vi "Package Typed Message.vi"(8 "error in (no error)":errorcluster, 11 "Group BOOL in":refnum<class "Group BOOL.lvclass">) -> (0 "error out":errorcluster, 2 "Data Msg":refnum<class "Message.lvclass">, 3 "Group BOOL out":refnum<class "Group BOOL.lvclass">)   [LabVIEW 2020, in "Vecto.lvlib" / "Group BOOL.lvclass"]
uses:
  Group BOOL.lvclass
  C:/dev/lv20CE/relink/lv-vecto/Vecto/Group/Group.lvclass
  lv-protoc/LV-Proto/Message/Message.lvclass
  Group/Group.lvclass/Group.ctl
  Group BOOL.lvclass/Group BOOL.ctl
  lv-volatus/messages/BoolData/Data.ctl
  Group Config/Group Config.lvclass/Group Config.ctl
  lv-volatus/messages/BoolData/Class/Msg.lvclass/Msg.ctl
  Double to Relative ns.vi
  lv-volatus/messages/BoolData/Class/Msg.lvclass
  C:/dev/lv20CE/relink/lv-protoc/LV-Proto/Message/Message.lvclass
  Group/Group.lvclass
  Group Config/Group Config.lvclass
  Vecto.lvlib
  lv-volatus/messages/BoolData/BoolData.lvlib
  C:/dev/lv20CE/relink/lv-vecto/Vecto/Group BOOL/Group BOOL.lvclass
  C:/dev/lv20CE/relink/lv-volatus/messages/BoolData/Class/Msg.lvclass
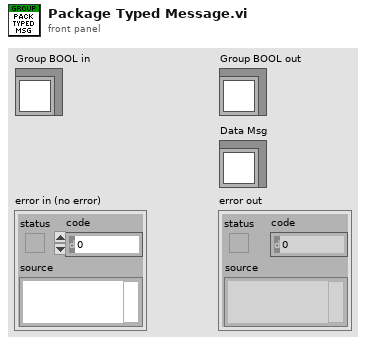
[diagram p1: front panel]
types:
  T1 = typedef "BoolData.lvlib/Data.ctl" = cluster{"group_name":string, "data_timestamp":i64, "scaled_data":bool[], "raw_data":bool[], "names_crc":u32}
  T2 = typedef "Vecto.lvlib/Group BOOL.lvclass/Ref.ctl" = cluster{"Scaled":bool[], "Timestamp":dbl[], "Raw":bool[]}
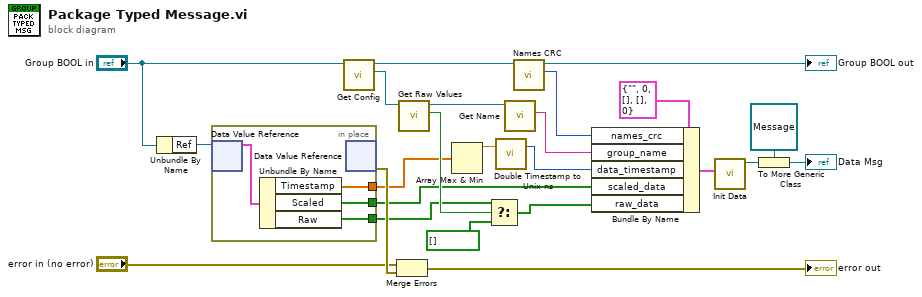
[diagram p0: block diagram]
diagram:
  n1 = Unbundle By Name("Group BOOL in") -> ("Ref"=w22:refnum<data-value>)
  n2 = in-place {
    in-place-border: [w27] -> w13
    in-place-border: [w26] -> w14
    in-place-border: [w25] -> w12
    n3 = in-place-dvr #1(w22) -> (w28:T2)  [unwired: 1 out]
    n4 = Unbundle By Name(w28) -> ("Timestamp"=w26:dbl[], "Scaled"=w27:bool[], "Raw"=w25:bool[])
    n5 = in-place-dvr #1() -> (w24:errorcluster)  [unwired: 1 in, 1 out]
  }
  n6 = call "Get Config.vi"("Group in"="Group BOOL in") -> ("Config"=w11:refnum<class "Group Config.lvclass">, "Group out"=w10:refnum<class "Group BOOL.lvclass">)  [unwired: 8 in, 1 out]
  n7 = Merge Errors("error in (no error)", w24) -> (→"error out":errorcluster)
  n8 = call "Get Raw Values.vi"("Group Config in"=w11) -> ("Raw Values"=w17:bool, "Group Config out"=w16:refnum<class "Group Config.lvclass">)  [unwired: 8 in, 1 out]
  n9 = Array Max & Min(array=w14) -> (max value=w21:dbl)  [unwired: 3 out]
  n10 = Select(t=w12, s=w17, f=bool[] []) -> (s? t:f=w18:bool[])
  n11 = call "Double Timestamp to Unix ns.vi"("Timestamp"=w21) -> ("unix ns"=w20:i64)  [unwired: 2 in]
  n12 = call "Get Name.vi"("Group Config in"=w16) -> ("Name"=w15:string)  [unwired: 8 in, 2 out]
  n13 = call "Names CRC.vi"("Group in"=w10) -> ("Names CRC"=w1:u32, "Group out"=→"Group BOOL out":refnum<class "Group BOOL.lvclass">)  [unwired: 9 in]
  n14 = Bundle By Name(cluster=T1 {"group_name"="", "data_timestamp"=0, "scaled_data"=[], "raw_data"=[], "names_crc"=0} ("BoolData"), "names_crc"=w1, "group_name"=w15, "data_timestamp"=w20, "scaled_data"=w13, "raw_data"=w18) -> (w7:T1)
  n15 = call "Init Data.vi"("Data"=w7) -> ("Msg out"=w6:refnum<class "Msg.lvclass">)  [unwired: 10 in]
  n16 = To More Generic Class(target class=refnum<class "Message.lvclass"> refnum ("Data Msg"), reference=w6) -> (generic class reference=→"Data Msg":refnum<class "Message.lvclass">)
